vi "InitGlobals.vi"   [LabVIEW 2014]
uses:
  <vilib>/Rock Robotics/WPI/Camera/WPI_CameraImageSize.ctl
  <vilib>/Rock Robotics/WPI/DriverStation/WPI_DriverStationRobotMode2.ctl
  Robot Global Data.vi
types:
  T1 = typedef "WPI_DriverStationRobotMode2.ctl" = enum16{"Autonomous Disabled", "Autonomous Enabled", "Teleop Disabled", "Teleop Enabled", "Disconnected", "Finish", "Test Disabled", "Test Enabled", "Emergency Stopped"}
  T2 = typedef "WPI_CameraImageSize.ctl" = enum16{"640x480", "320x240", "160x120", "Custom"}
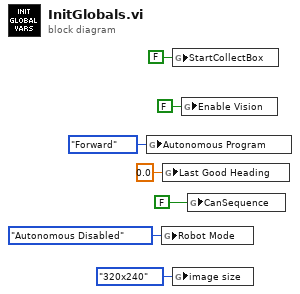
[diagram p0: block diagram]
diagram:
  n1 = global write "Robot Global Data.vi" "Autonomous Program"(enum16{"Forward", "Stack", "Null"}."Forward" ("Autonomous Program")) -> ()
  n2 = global write "Robot Global Data.vi" "Robot Mode"(WPI_DriverStationRobotMode2."Autonomous Disabled" ("Robot Mode")) -> ()
  n3 = global write "Robot Global Data.vi" "Last Good Heading"(0.0 ("Last Good Heading")) -> ()
  n4 = global write "Robot Global Data.vi" "StartCollectBox"(FALSE ("StartCollectBox")) -> ()
  n5 = global write "Robot Global Data.vi" "image size"(WPI_CameraImageSize."320x240" ("image size")) -> ()
  n6 = global write "Robot Global Data.vi" "Enable Vision"(FALSE ("Enable Vision")) -> ()
  n7 = global write "Robot Global Data.vi" "CanSequence"(FALSE ("Last Toggle State")) -> ()
